vi "NI VeriStand - Get Parameter 2D Array Values.vi"(7 "Target":string, 8 "error in (no error)":errorcluster, 10 "Parameter":string, 11 "ModelManager in":T1) -> (0 "error out":errorcluster, 2 "Values":dbl[][](array[numeric]), 3 "ModelManager out":T1)   [LabVIEW 2020, in "NI_VS ModelManager ExecutionAPI.lvlib"]
doc: "Returns values of model parameters present on the target. You must manually select the polymorphic instance to use."
uses:
  <vilib>/NI VeriStand/Execution/ModelManager/NI_VS ModelManager ExecutionAPI.lvlib
  <vilib>/NI VeriStand/Execution/ModelManager/ModelManagerAPI.ctl
  NationalInstruments.VeriStand.ClientAPI
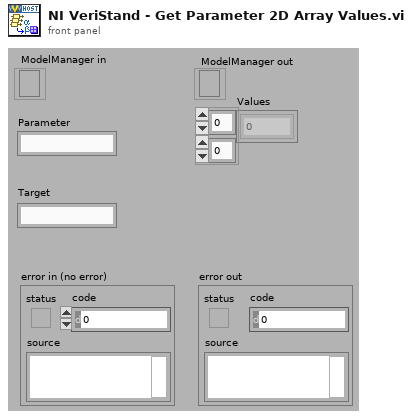
[diagram p1: front panel]
types:
  T1 = typedef "NI_VS ModelManager ExecutionAPI.lvlib/ModelManagerAPI.ctl" = refnum<k24>
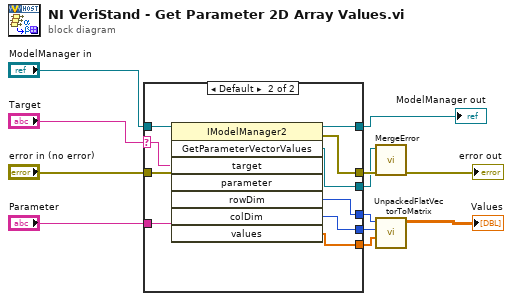
[diagram p0: block diagram]
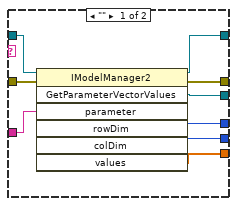
[diagram p2: hidden frame]
diagram:
  n1 = case shown="Default" "Target" {
    selector: "Target" -> [_ w22]
    tunnel: "ModelManager in" -> [w21 w31]
    tunnel: [w20 w30] -> w11
    tunnel: [w19 w29] -> w10
    tunnel: [w18 w28] -> w9
    tunnel: "error in (no error)" -> [w17 w27]
    tunnel: "Parameter" -> [w16 w26]
    tunnel: [w15 w23] -> w5
    tunnel: [w14 w24] -> w4
    tunnel: [w13 w25] -> w3
    frame "" {
      n2 = invoke class="IModelManager2" method="GetParameterVectorValues"(reference=w21, error in=w17, "parameter"=w16) -> (reference out=w20:T1, error out=w19:errorcluster, "GetParameterVectorValues"=w18:refnum<k24>, "rowDim"=w15:u32, "colDim"=w14:u32, "values"=w13:dbl[])  [unwired: 4 in, 1 out]
    }
    frame Default {
      n3 = invoke class="IModelManager2" method="GetParameterVectorValues"(reference=w31, error in=w27, "target"=w22, "parameter"=w26) -> (reference out=w30:T1, error out=w29:errorcluster, "GetParameterVectorValues"=w28:refnum<k24>, "rowDim"=w23:u32, "colDim"=w24:u32, "values"=w25:dbl[])  [unwired: 4 in, 2 out]
    }
  }
  "ModelManager out" <- w11
  n4 = call <vilib>:"MergeError.vi"("error in (no error)"=w10, "Error"=w9) -> ("error out"=→"error out":errorcluster)  [unwired: 9 out]
  n5 = call <vilib>:"UnpackedFlatVectorToMatrix.vi"("FlatValues"=w3, "colDim"=w4, "rowDim"=w5) -> ("Matrix"=→"Values":dbl[][])  [unwired: 8 out]
